vi "Initialize.vi"(8 "error in (no error)":errorcluster, 11 "PSP-405 resource in":refnum<visa-resource-name>) -> (0 "error out":errorcluster, 3 "PSP-405 resource out":refnum<visa-resource-name>)   [LabVIEW 2017, in "GW Instek PSP-405.lvlib"]
doc: "Establishes communication with the instrument. Therefore, call this VI before calling other instrument driver VIs for this instrument. Generally, you need to call the <B>Initialize VI</B> only once at the beginning of an application."
uses:
  GW Instek PSP-405.lvlib
  <vilib>/Instr/_visa.llb/VISA Configure Serial Port (Instr).vi
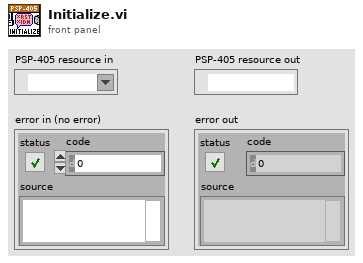
[diagram p1: front panel]
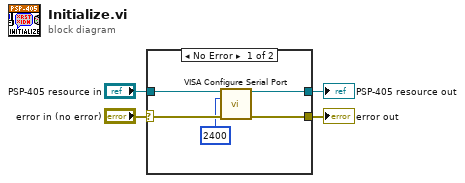
[diagram p0: block diagram]
diagram:
  n1 = case shown="No Error" "error in (no error)" {
    selector: "error in (no error)" -> [w9 w11]
    tunnel: "PSP-405 resource in" -> [w8 w10]
    tunnel: [w6 w11] -> w2
    tunnel: [w5 w10] -> w1
    frame No Error {
      n2 = call-poly "VISA Configure Serial Port"("VISA resource name"=w8, "baud rate (9600)"=u32 2400, "error in (no error)"=w9) -> ("VISA resource name out"=w5:refnum<visa-resource-name>, "error out"=w6:errorcluster)  [unwired: 11 in]
    }
    frame Error {
    }
  }
  "error out" <- w2
  "PSP-405 resource out" <- w1
